vi "ADAM_health_subpanel_20190329.vi"() -> ()   [LabVIEW 2018]
uses:
  health_state.ctl
  health_Loop_Clust.ctl
  Epimedia_Connex_Source/Controls/Enums/WatchdogTimer_Enum.ctl
  Epimedia_Connex_Source/HDF5/HDF5_ADAM_Data.ctl
  Epimedia_Connex_Source/Controls/Enums/LogLoopEnum.ctl
panel:
  out "Chart":T1(graph)
  out "Enum":T2
  out "error out":errorcluster
  in  "error in":errorcluster
  out "Hatch Command":bool
  in  "Sample Now":bool
  out "Faults Since":string
  out "Total Faults":i16
  out "Running LED":bool
  out "Progress Bar":dbl(slide) scale=0.0..60.0
  out "Error Dialog":string="Error Message Display Box"
  out "Faults":bool[](array[boolean])
  in  "Toggle Hatch":bool
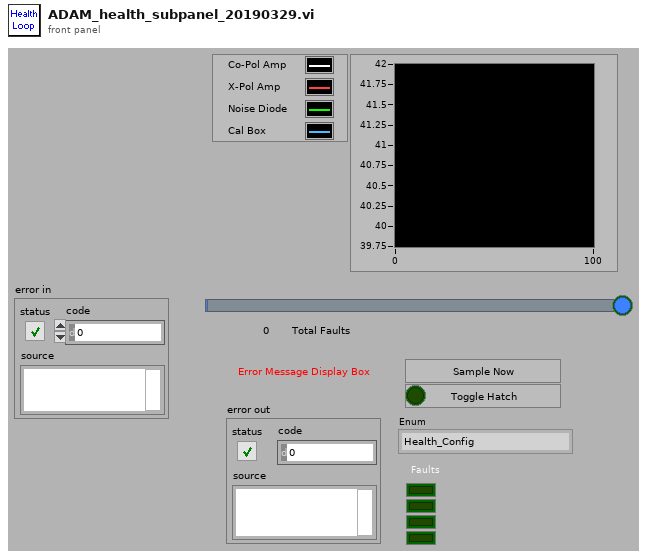
[diagram p1: front panel]
types:
  T1 = cluster{"[0]":dbl, "[1]":dbl, "[2]":dbl, "[3]":dbl}
  T2 = typedef "health_state.ctl" = enum16{"Health_Config", "Health_Wait", "Health_Read", "Health_Log", "Health_Exit"}
  T3 = typedef "health_Loop_Clust.ctl" = cluster{"nSignals":i32, "logname":string, "time":timestamp, "dir":path, "adamSerial":cluster{"port":refnum<visa-resource-name>, "timeout":u32, "baud":u32, "dataBits":u16, "stopBits":u16, "flowControl":u16, "parity":u16, "termChar":bool, "checkSum":bool}, "fiberSerial":cluster{"port1":refnum<visa-resource-name>, "port2":refnum<visa-resource-name>, "timeout":u32, "baud":u32, "dataBits":u16, "stopBits":u16, "flowControl":u16, "parity":u16, "termChar":bool, "checkSum":bool, "fiber1On":bool, "fiber2On":bool}, "signal":cluster{"src":enum16{"adam", "fiber", "te"}[], "id":string[], "ch":string[], "descrip":string[], "units":string[], "scale":dbl[], "hi":dbl[], "lo":dbl[], "rec":bool[], "fault":bool[], "val":dbl[]}, "teSerial":cluster{"port":refnum<visa-resource-name>, "timeout":u32, "baud":u32, "dataBits":u16, "stopBits":u16, "flowControl":u16, "parity":u16, "termChar":bool, "checkSum":bool, "checkSumVal":string}, "lograte":u32, "calSwitch":bool, "logoffset":dbl}
  T4 = typedef "WatchdogTimer_Enum.ctl" = enum16{"ResetAll", "CheckAll", "HW1", "HW2", "Tones", "FP", "Noise", "Log", "TCP", "AI", "TC", "ADAM", "Disdrom", "TE", "Weather"}
  T5 = typedef "HDF5_ADAM_Data.ctl" = cluster{"Timestamp":dbl, "Time string":string, "Fault 1":bool, "Fault 2":bool, "Fault 3":bool, "Fault 4":bool, "Fault 5":bool, "Fault 6":bool, "Value 1":dbl, "Value 2":dbl, "Value 3":dbl, "Value 4":dbl, "Value 5":dbl, "Value 6":dbl}
  T6 = cluster{"port":refnum<visa-resource-name>, "timeout":u32, "baud":u32, "dataBits":u16, "stopBits":u16, "flowControl":u16, "parity":u16, "termChar":bool, "checkSum":bool}
  T7 = typedef "LogLoopEnum.ctl" = enum16{"Log_Init", "Log_Config", "Log_CfgAlarm", "Log_TimeDomain", "Log_Tone", "Log_NoiseTrace", "Log_NoiseSum", "Log_DO", "Log_AI", "Log_TC", "Log_Disdrom", "Log_Weather", "Log_TE", "Log_ADAM", "Log_UPS", "Log_ChkTime", "Log_Alarm", "Log_SSH", "Log_Write", "Log_Exit"}
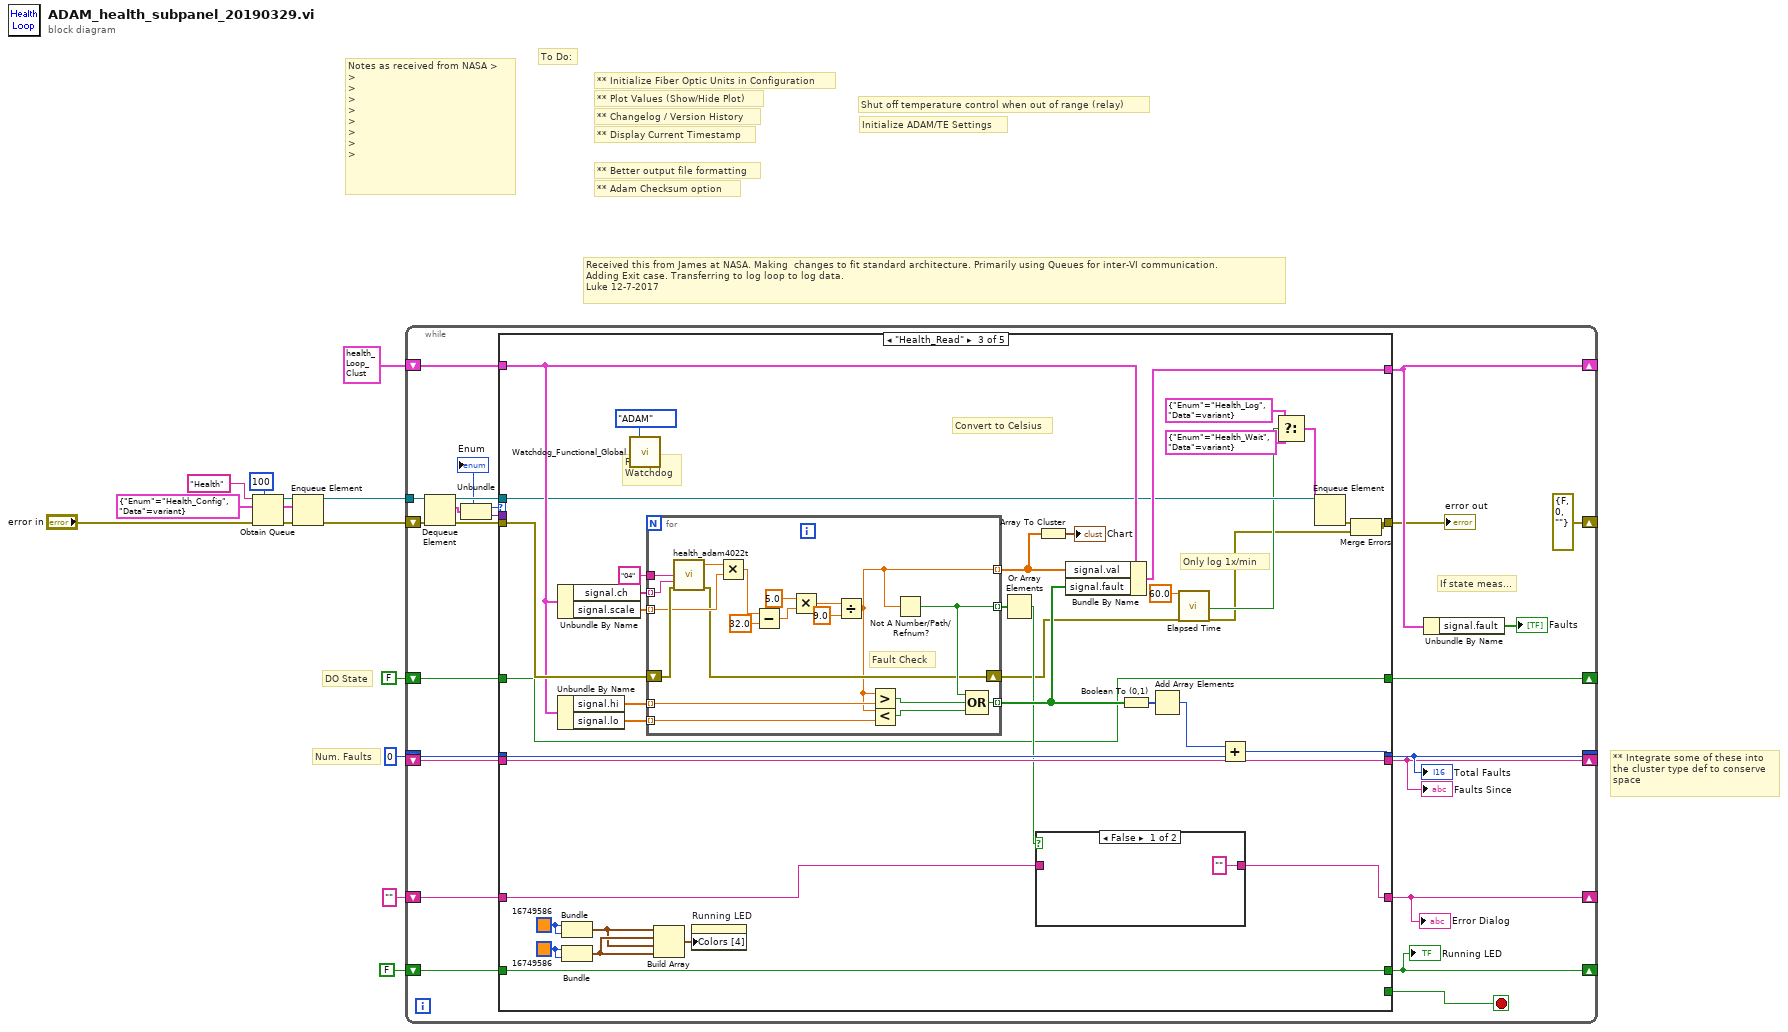
[diagram p0: block diagram]
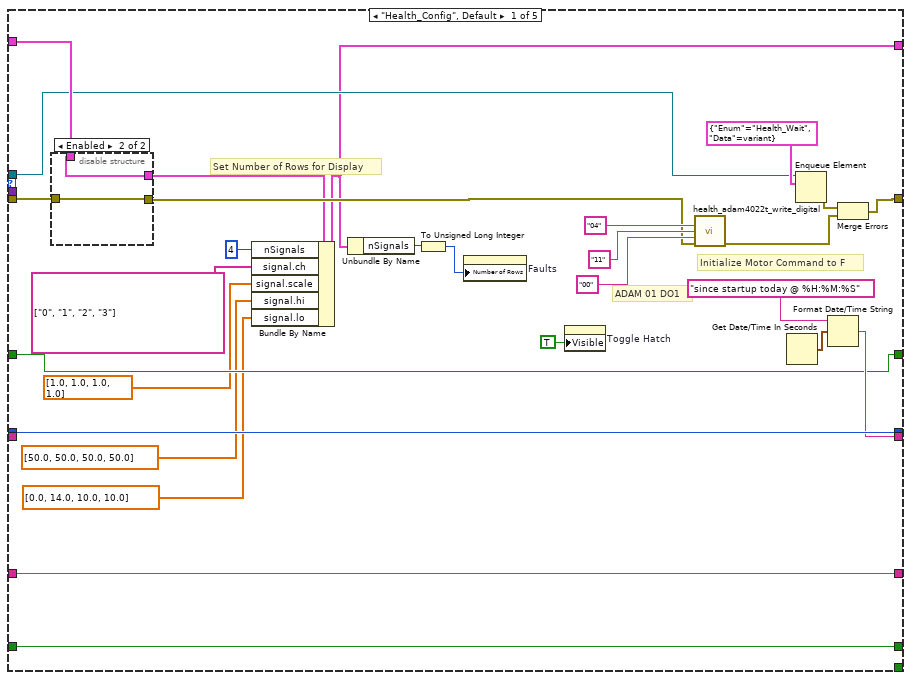
[diagram p2: hidden frame]
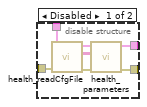
[diagram p3: hidden frame]
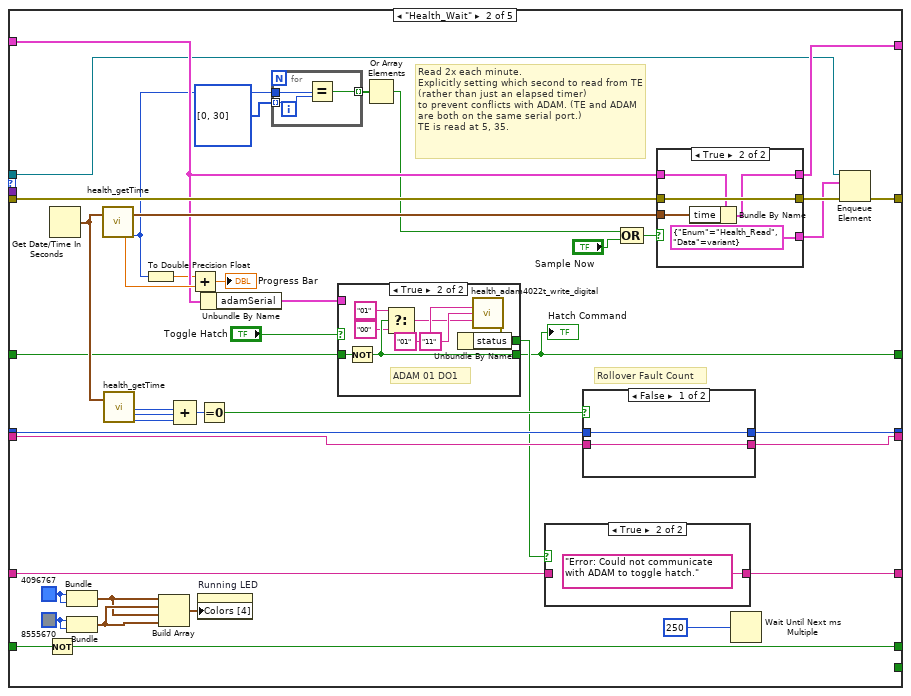
[diagram p4: hidden frame]
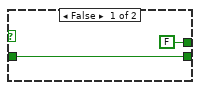
[diagram p6: hidden frame]
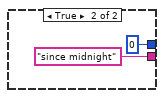
[diagram p7: hidden frame]
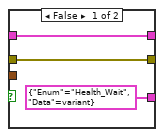
[diagram p8: hidden frame]
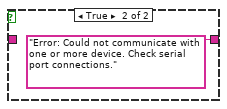
[diagram p9: hidden frame]
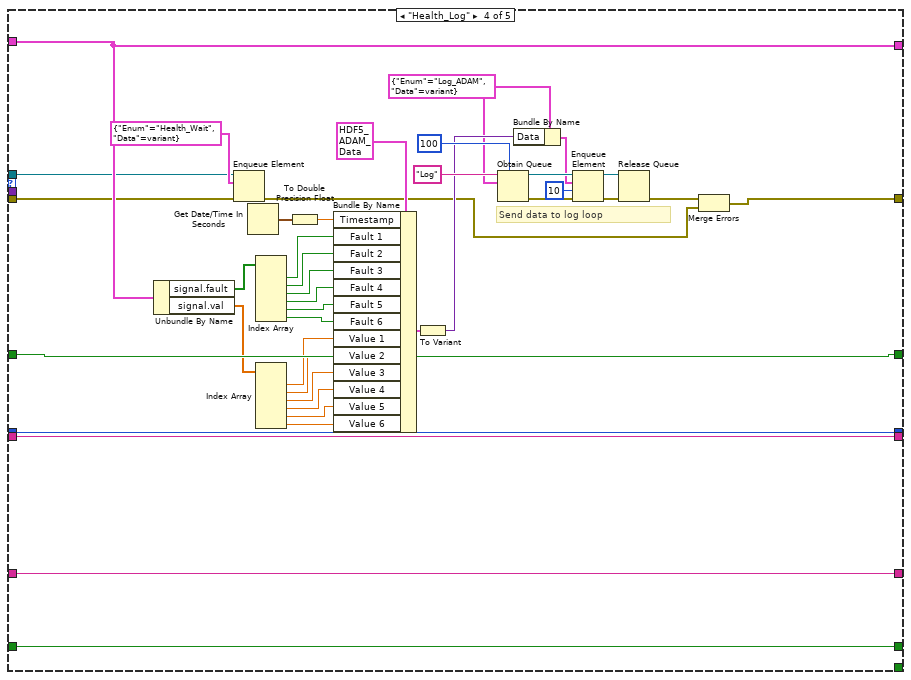
[diagram p10: hidden frame]
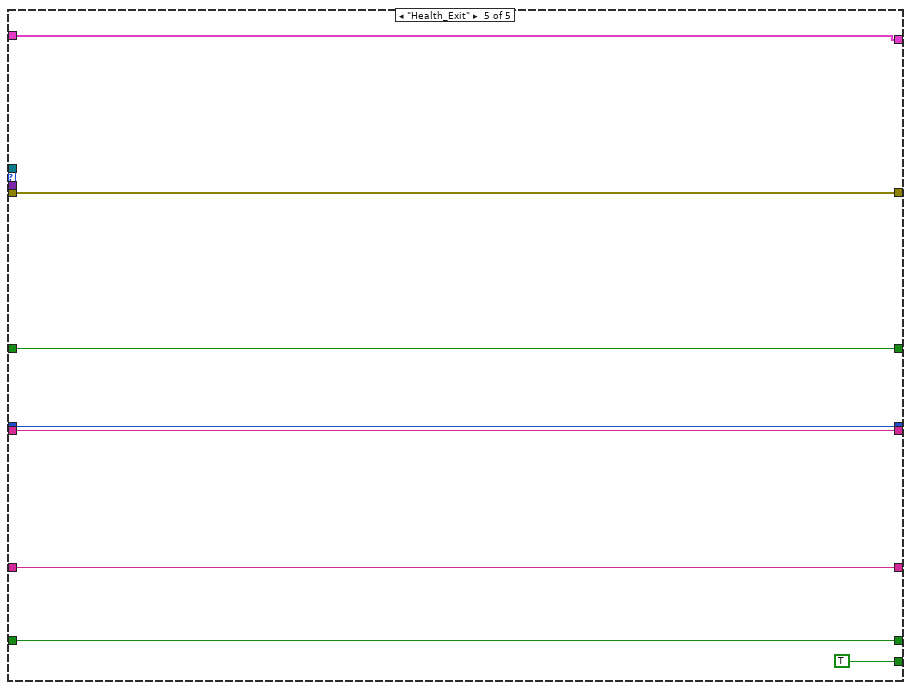
[diagram p11: hidden frame]
diagram:
  w4 = cluster{"Enum":T2, "Data":variant} {"Enum"=enum."Health_Config", "Data"=variant}
  # "Notes as received from NASA >\n>\n>\n>\n>\n>\n>\n>\n>"
  # "Received this from James at NASA. Making  changes to fit standard architecture. Primarily using Queues for inter-VI communication.\nAdding Exit case. Transferring to log loop to log data.\nLuke 12-7-2017"
  # "DO State"
  # "Initialize ADAM/TE Settings"
  # "Shut off temperature control when out of range (relay)"
  # "** Integrate some of these into\nthe cluster type def to conserve\nspace"
  # "** Changelog / Version History"
  # "** Plot Values (Show/Hide Plot)"
  # "** Display Current Timestamp"
  # "** Adam Checksum option"
  # "Num. Faults"
  # "** Better output file formatting"
  # "To Do:"
  # "** Initialize Fiber Optic Units in Configuration"
  n1 = Obtain Queue(max queue size (-1, unlimited)=100, name (unnamed)="Health", element data type=w4, error in (no error)="error in") -> (queue out=w6:refnum<queue>, error out=w5:errorcluster)  [unwired: 1 in, 1 out]
  n2 = Enqueue Element(queue=w6, element=w4, error in (no error)=w5) -> (queue out=w1:refnum<queue>, error out=w3:errorcluster)  [unwired: 1 in, 1 out]
  n3 = while {
    shift-right: [w33] -> _
    shift-left: T3 {"nSignals"=0, "logname"="", "time"=timestamp(0 s since 1904-01-01), "dir"=path "", "adamSerial"={"port"="", "timeout"=0, "baud"=0, "dataBits"=0, "stopBits"=0, "flowControl"=0, "parity"=0, "termChar"=FALSE, "checkSum"=FALSE}, "fiberSerial"={"port1"="", "port2"="", "timeout"=0, "baud"=0, "dataBits"=0, "stopBits"=0, "flowControl"=0, "parity"=0, "termChar"=FALSE, "checkSum"=FALSE, "fiber1On"=FALSE, "fiber2On"=FALSE}, "signal"={"src"=[], "id"=[], "ch"=[], "descrip"=[], "units"=[], "scale"=[], "hi"=[], "lo"=[], "rec"=[], "fault"=[], "val"=[]}, "teSerial"={"port"="", "timeout"=0, "baud"=0, "dataBits"=0, "stopBits"=0, "flowControl"=0, "parity"=0, "termChar"=FALSE, "checkSum"=FALSE, "checkSumVal"=""}, "lograte"=0, "calSwitch"=FALSE, "logoffset"=0.0} ("hDout") -> [w36]
    shift-right: [errorcluster {"status"=FALSE, "code"=0, "source"=""} ("error out")] -> _
    shift-left: w3 -> [w23]
    shift-right: [w34] -> _
    shift-left: FALSE -> [w35]
    shift-right: [w30] -> _
    shift-left: i16 0 -> [w31]
    shift-right: [w29] -> _
    shift-left: _ -> [w28]
    shift-right: [w27] -> _
    shift-left: "" ("Error Dialog") -> [w26]
    shift-right: [w25] -> _
    shift-left: FALSE -> [w24]
    tunnel: w1 -> [w21]
    stop <- w16 stop-if-true
    # "If state meas..."
    n4 = Dequeue Element(queue=w21, error in (no error)=w23) -> (queue out=w20:refnum<queue>, element=w19:cluster{"Enum":T2, "Data":variant}, error out=w22:errorcluster)  [unwired: 1 in, 1 out]
    n5 = Unbundle(w19) -> ("Enum"=w18:T2, "Data"=w17:variant)
    "Enum" <- w18
    n6 = case shown="\"Health_Read\"" w18 {
      tunnel: w22 -> [w64 w101 w172 w233 w248]
      tunnel: [w45 w102 w173 w239 w247] -> w33
      tunnel: w36 -> [w63 w87 w162 w239 w247]
      tunnel: [w62 w110 w179 w240 w242] -> w34
      tunnel: w35 -> [w62 w111 w179 w240 w242]
      tunnel: [w60 w96 w166 w238 w245] -> w30
      tunnel: w31 -> [w60 w95 w165 w238 w245]
      tunnel: [w58 w94 w161 w237 w244] -> w29
      tunnel: w28 -> [_ w93 w161 w237 w244]
      tunnel: [w56 w85 w159 w236 w243] -> w27
      tunnel: w26 -> [w56 w84 w157 w236 w243]
      tunnel: [w39 w80 w144 w201 w248] -> w15
      tunnel: [w55 w82 w156 w235 w246] -> w25
      tunnel: w24 -> [w55 w88 w156 w235 w246]
      tunnel: w20 -> [w47 w79 w155 w232 _]
      tunnel: w17 -> [_ _ _ _ _]
      tunnel: [_ _ _ _ TRUE ("stop")] -> w16
      frame "Health_Config", Default {
        # "Initialize Motor Command to F"
        # "ADAM 01 DO1"
        # "Set Number of Rows for Display"
        n7 = disable-structure shown="Enabled" {
          disable-tunnel: w64 -> [w70 w72]
          disable-tunnel: w63 -> [w67 w71]
          disable-tunnel: [w66 w71] -> w46
          disable-tunnel: [w65 w72] -> w49
          frame Disabled {
            n8 = call "health_readCfgFile.vi"("error in \n(no error)"=w70) -> ("error out"=w68:errorcluster, "parameters"=w69:string[][])  [unwired: 9 in]
            n9 = call "health_parameters.vi"("error in\n(no error)"=w68, "parameters"=w69, "hDin"=w67) -> ("error out"=w65:errorcluster, "hDout"=w66:T3)  [unwired: 7 in]
          }
          frame Enabled {
          }
        }
        n10 = Bundle By Name(cluster=w46, "nSignals"=4, "signal.ch"=string[] ["0", "1", "2", "3"], "signal.scale"=dbl[] [1.0, 1.0, 1.0, 1.0], "signal.hi"=dbl[] [50.0, 50.0, 50.0, 50.0], "signal.lo"=dbl[] [0.0, 14.0, 10.0, 10.0]) -> (w45:T3)
        n11 = Unbundle By Name(w45) -> ("nSignals"=w54:i32)
        n12 = To Unsigned Long Integer(number=w54) -> (unsigned 32bit integer=w61:u32)
        n13 = property on="Faults" class="Arr (strict)"("Number of Rows"=w61) -> ()  [unwired: 2 in, 2 out]
        n14 = property on="Toggle Hatch" class="Bool"("Visible"=TRUE) -> ()  [unwired: 2 in, 2 out]
        n15 = call "health_adam4022t_write_digital.vi"("Address"="04", "Channel"="11", "Value"="00" ("Address"), "Error In"=w49) -> ("Error Out"=w37:errorcluster)  [unwired: 9 in, 2 out]
        n16 = Get Date/Time In Seconds() -> (seconds since 1Jan1904=w57:timestamp)
        n17 = Enqueue Element(queue=w47, element=cluster{"Enum":T2, "Data":variant} {"Enum"=enum."Health_Wait", "Data"=variant}) -> (error out=w38:errorcluster)  [unwired: 2 in, 2 out]
        n18 = Format Date/Time String(time format string (%c)="since startup today @ %H:%M:%S", seconds (now)=w57) -> (date/time string=w58:string)  [unwired: 1 in]
        n19 = Merge Errors(w38, w37) -> (w39:errorcluster)
      }
      frame "Health_Wait" {
        w108 = u32 8555670
        w107 = u32 4096767
        # "Read 2x each minute.\nExplicitly setting which second to read from TE (rather than just an elapsed timer)\nto prevent conflicts with ADAM. (TE and ADAM are both on the same serial port.)\nTE is read at 5, 35."
        # "Rollover Fault Count"
        n20 = Not(x=w111) -> (.not. x?=w110:bool)
        n21 = Get Date/Time In Seconds() -> (seconds since 1Jan1904=w92:timestamp)
        n22 = Bundle(w107, w107) -> (w105:cluster{u32, u32})  [unwired: 1 in]
        n23 = Bundle(w108, w108) -> (w106:cluster{u32, u32})  [unwired: 1 in]
        n24 = call "health_getTime.vi"("Current Time"=w92) -> ("Fractional Seconds"=w104:dbl, "Seconds"=w75:u32)  [unwired: 11 in, 6 out]
        n25 = call "health_getTime.vi"("Current Time"=w92) -> ("Hour"=w98:u32, "Minutes"=w99:u32, "Seconds"=w100:u32)  [unwired: 11 in, 5 out]
        n26 = To Double Precision Float(number=w75) -> (double precision float=w73:dbl)
        n27 = Build Array(w105, w106, w105, w106) -> (w109:cluster{u32, u32}[])
        n28 = Compound Arithmetic op=ADD(w98, w99, w100) -> (w112:u32)
        n29 = Add(x=w73, y=w104) -> (x+y=→"Progress Bar":dbl)
        n30 = property on="Running LED" class="Bool (strict)"("Colors [4]"=w109) -> ()  [unwired: 2 in, 2 out]
        n31 = Equal To 0?(x=w112) -> (x = 0?=w97:bool)
        n32 = Unbundle By Name(w87) -> ("adamSerial"=w86:T6)
        n33 = for {
          tunnel: w75 -> [w116]
          tunnel: u32[] [0, 30] ("y") -> [w115] mode=indexing
          tunnel: [w114] -> w77 mode=indexing
          n34 = Equal?(x=w116, y=w115) -> (x = y?=w114:bool)
        }
        n35 = case shown="True" "Toggle Hatch" {
          tunnel: [w120 w128] -> w82
          tunnel: w88 -> [w120 w129]
          tunnel: w86 -> [_ _]
          tunnel: [FALSE ("status") w127] -> w83
          frame False {
          }
          frame True {
            # "ADAM 01 DO1"
            n36 = Not(x=w129) -> (.not. x?=w128:bool)
            n37 = Select(t="01" ("Address"), s=w128, f="00" ("Address")) -> (s? t:f=w121:string)
            n38 = call "health_adam4022t_write_digital.vi"("Address"="01", "Channel"="11", "Value"=w121) -> ("Error Out"=w124:errorcluster)  [unwired: 10 in, 2 out]
            n39 = Unbundle By Name(w124) -> ("status"=w127:bool)
          }
        }
        "Hatch Command" <- w82
        n40 = Or Array Elements(Boolean array=w77) -> (logical OR=w74:bool)
        n41 = case shown="True" w83 {
          tunnel: [w117 "Error: Could not communicate with ADAM to toggle hatch." ("Error Dialog")] -> w85
          tunnel: w84 -> [w117 _]
          frame False {
          }
          frame True {
          }
        }
        n42 = case shown="False" w97 {
          tunnel: [w131 i16 0] -> w96
          tunnel: w95 -> [w131 _]
          tunnel: [w130 "since midnight" ("time format string (%c)")] -> w94
          tunnel: w93 -> [w130 _]
          frame False {
          }
          frame True {
          }
        }
        n43 = Compound Arithmetic op=OR(w74, "Sample Now") -> (w90:bool)
        n44 = case shown="True" w90 {
          tunnel: [cluster{"Enum":T2, "Data":variant} {"Enum"=enum."Health_Wait", "Data"=variant} cluster{"Enum":T2, "Data":variant} {"Enum"=enum."Health_Read", "Data"=variant}] -> w78
          tunnel: [w136 w138] -> w102
          tunnel: w87 -> [w136 w140]
          tunnel: [w135 w141] -> w81
          tunnel: w101 -> [w135 w141]
          tunnel: w92 -> [_ w139]
          frame False {
          }
          frame True {
            n45 = Bundle By Name(cluster=w140, "time"=w139) -> (w138:T3)
          }
        }
        n46 = Wait Until Next ms Multiple(millisecond multiple=u32 250 ("milliseconds to wait")) -> ()  [unwired: 1 out]
        n47 = Enqueue Element(queue=w79, element=w78, error in (no error)=w81) -> (error out=w80:errorcluster)  [unwired: 1 in, 2 out]
      }
      frame "Health_Read" {
        w178 = u32 16749586
        w177 = u32 16749586
        # "Reset\nWatchdog"
        # "Only log 1x/min"
        # "Convert to Celsius"
        n48 = Unbundle By Name(w162) -> ("signal.ch"=w164:string[], "signal.scale"=w163:dbl[])
        n49 = Unbundle By Name(w162) -> ("signal.hi"=w171:dbl[], "signal.lo"=w170:dbl[])
        n50 = Bundle(w177, w177) -> (w175:cluster{u32, u32})  [unwired: 1 in]
        n51 = Bundle(w178, w178) -> (w176:cluster{u32, u32})  [unwired: 1 in]
        n52 = call "Watchdog_Functional_Global.vi"("Watchdog"=WatchdogTimer_Enum."ADAM") -> ()  [unwired: 8 in, 3 out]
        n53 = for {
          tunnel: w164 -> [w200] mode=indexing
          tunnel: [w182] -> w147 mode=indexing
          tunnel: w171 -> [w199] mode=indexing
          tunnel: w170 -> [w198] mode=indexing
          tunnel: [w195] -> w169 mode=indexing
          tunnel: w163 -> [w193] mode=indexing
          tunnel: [w192] -> w160 mode=indexing
          shift-right: [w191] -> w153
          shift-left: w172 -> [w194]
          tunnel: "04" ("Address") -> [w189]
          # "Fault Check"
          n54 = call "health_adam4022t.vi"("Address"=w189, "Channel"=w200, "Error In"=w194) -> ("Value"=w190:dbl, "Error Out"=w191:errorcluster)  [unwired: 11 in]
          n55 = Multiply(x=w190, y=w193) -> (x*y=w183:dbl)
          n56 = Subtract(x=w183, y=32.0) -> (x-y=w187:dbl)
          n57 = Multiply(x=5.0, y=w187) -> (x*y=w186:dbl)
          n58 = Divide(x=w186, y=9.0) -> (x/y=w182:dbl)
          n59 = Greater?(x=w182, y=w199) -> (0:w197:bool)
          n60 = Less?(x=w182, y=w198) -> (x < y?=w196:bool)
          n61 = Not A Number/Path/Refnum?(number/path/refnum=w182) -> (NaN/Path/Refnum?=w192:bool)
          n62 = Compound Arithmetic op=OR(w192, w197, w196) -> (w195:bool)
        }
        n63 = Build Array(w175, w176, w175, w176) -> (w174:cluster{u32, u32}[])
        n64 = property on="Running LED" class="Bool (strict)"("Colors [4]"=w174) -> ()  [unwired: 2 in, 2 out]
        n65 = Or Array Elements(Boolean array=w160) -> (logical OR=w158:bool)
        n66 = case shown="False" w158 {
          tunnel: ["" ("Error Dialog") "Error: Could not communicate with one or more device. Check serial port connections." ("Error Dialog")] -> w159
          tunnel: w157 -> [_ _]
          frame False {
          }
          frame True {
          }
        }
        n67 = Array To Cluster(array=w147) -> (cluster=→"Chart":T1)
        n68 = Bundle By Name(cluster=w162, "signal.val"=w147, "signal.fault"=w169) -> (w173:T3)
        n69 = Boolean To (0,1)(Boolean=w169) -> (0, 1=w167:i16[])
        n70 = Add Array Elements(numeric array=w167) -> (sum=w168:i16)
        n71 = call "Elapsed Time"("Time Target (s)"=60.0, "error in (no error)"=w153) -> ("Time has Elapsed"=w148:bool, "error out"=w143:errorcluster)  [unwired: 10 in, 6 out]
        n72 = Add(x=w168, y=w165) -> (x+y=w166:i16)
        n73 = Select(t=cluster{"Enum":T2, "Data":variant} {"Enum"=enum."Health_Log", "Data"=variant}, s=w148, f=cluster{"Enum":T2, "Data":variant} {"Enum"=enum."Health_Wait", "Data"=variant}) -> (s? t:f=w149:cluster{"Enum":T2, "Data":variant})
        n74 = Enqueue Element(queue=w155, element=w149) -> (error out=w145:errorcluster)  [unwired: 2 in, 2 out]
        n75 = Merge Errors(w145, w143) -> (w144:errorcluster)
      }
      frame "Health_Log" {
        w207 = cluster{"Enum":T7, "Data":variant} {"Enum"=enum."Log_ADAM", "Data"=variant}
        # "Send data to log loop"
        n76 = Unbundle By Name(w239) -> ("signal.fault"=w229:bool[], "signal.val"=w231:dbl[])
        n77 = Enqueue Element(queue=w232, element=cluster{"Enum":T2, "Data":variant} {"Enum"=enum."Health_Wait", "Data"=variant}, error in (no error)=w233) -> (error out=w202:errorcluster)  [unwired: 1 in, 2 out]
        n78 = Get Date/Time In Seconds() -> (seconds since 1Jan1904=w204:timestamp)
        n79 = Index Array(array=w229) -> (element #1=w228:bool, element #2=w227:bool, element #3=w226:bool, element #4=w225:bool, element #5=w224:bool, element #6=w223:bool)  [unwired: 6 in]
        n80 = Index Array(array=w231) -> (element #1=w222:dbl, element #2=w221:dbl, element #3=w220:dbl, element #4=w219:dbl, element #5=w218:dbl, element #6=w217:dbl)  [unwired: 6 in]
        n81 = To Double Precision Float(number=w204) -> (double precision float=w205:dbl)
        n82 = Bundle By Name(cluster=T5 {"Timestamp"=0.0, "Time string"="", "Fault 1"=FALSE, "Fault 2"=FALSE, "Fault 3"=FALSE, "Fault 4"=FALSE, "Fault 5"=FALSE, "Fault 6"=FALSE, "Value 1"=0.0, "Value 2"=0.0, "Value 3"=0.0, "Value 4"=0.0, "Value 5"=0.0, "Value 6"=0.0}, "Timestamp"=w205, "Fault 1"=w228, "Fault 2"=w227, "Fault 3"=w226, "Fault 4"=w225, "Fault 5"=w224, "Fault 6"=w223, "Value 1"=w222, "Value 2"=w221, "Value 3"=w220, "Value 4"=w219, "Value 5"=w218, "Value 6"=w217) -> (w209:T5)
        n83 = To Variant(anything=w209) -> (Variant=w208:variant)
        n84 = Obtain Queue(max queue size (-1, unlimited)=100, name (unnamed)="Log", element data type=w207) -> (queue out=w214:refnum<queue>, error out=w213:errorcluster)  [unwired: 2 in, 1 out]
        n85 = Bundle By Name(cluster=w207, "Data"=w208) -> (w212:cluster{"Enum":T7, "Data":variant})
        n86 = Enqueue Element(queue=w214, element=w212, timeout in ms (-1)=10, error in (no error)=w213) -> (queue out=w211:refnum<queue>, error out=w210:errorcluster)  [unwired: 1 out]
        n87 = Release Queue(queue=w211, error in (no error)=w210) -> (error out=w203:errorcluster)  [unwired: 1 in, 2 out]
        n88 = Merge Errors(w203, w202) -> (w201:errorcluster)
      }
      frame "Health_Exit" {
      }
    }
    "Running LED" <- w34
    "Total Faults" <- w30
    "Faults Since" <- w29
    "Error Dialog" <- w27
    "error out" <- w15
    n89 = Unbundle By Name(w33) -> ("signal.fault"=→"Faults":bool[])
  }
